vi "CorrelImages.vi"   [LabVIEW 2014]
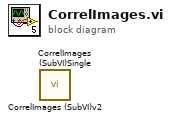
[diagram p0: block diagram]
diagram:
  n1 = call "CorrelImages (SubVI)v2.vi"() -> ()  [unwired: 8 in, 4 out]
  n2 = call "CorrelImages (SubVI)Single.vi"() -> ()  [unwired: 8 in, 4 out]
